vi "ExNframeBigBufNoDisplay.vi"() -> ()   [LabVIEW 2010]
uses:
  Open-Close Hardware/CamHandle.vi
panel:
  in  "Path":path=path "C:/Users/Public/Documents/SItoolkit/LabVIEW/Data Files/nframe.spe"
  in  "Number of Images":u32=1000 min=1 step=1
  out "ready to \nstart":bool
  in  "Start collection":bool
  in  "Exposure":dbl=1e-05 min=0.0 step=1e-06 format="%.7f"
  out "error out":errorcluster
  in  "error in (no error)":errorcluster
  # "ExCircNframeBigBufNoDisplay:\nThis example collects,  and saves in \na .spe file the number of images selected. This \nexample requires the camera have circular \nbuffers capability. \nFirst this example creates an array of image \nhandles. It then collects data into this array.\nFinally it displays and saves all the images."
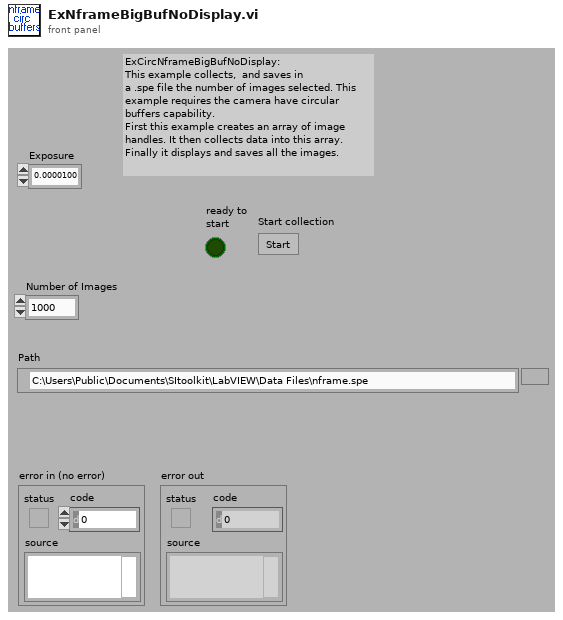
[diagram p1: front panel]
types:
  T1 = cluster{"acquire focus mode":u32, "Exposure":dbl, "Number of Images":u32, "Software accumulation":u32}
  T2 = cluster{"Camera Handle":u32, "Pulser Handle":u32, "File Handle":u32, "Display Handle":u32, "Image Handle":u32}
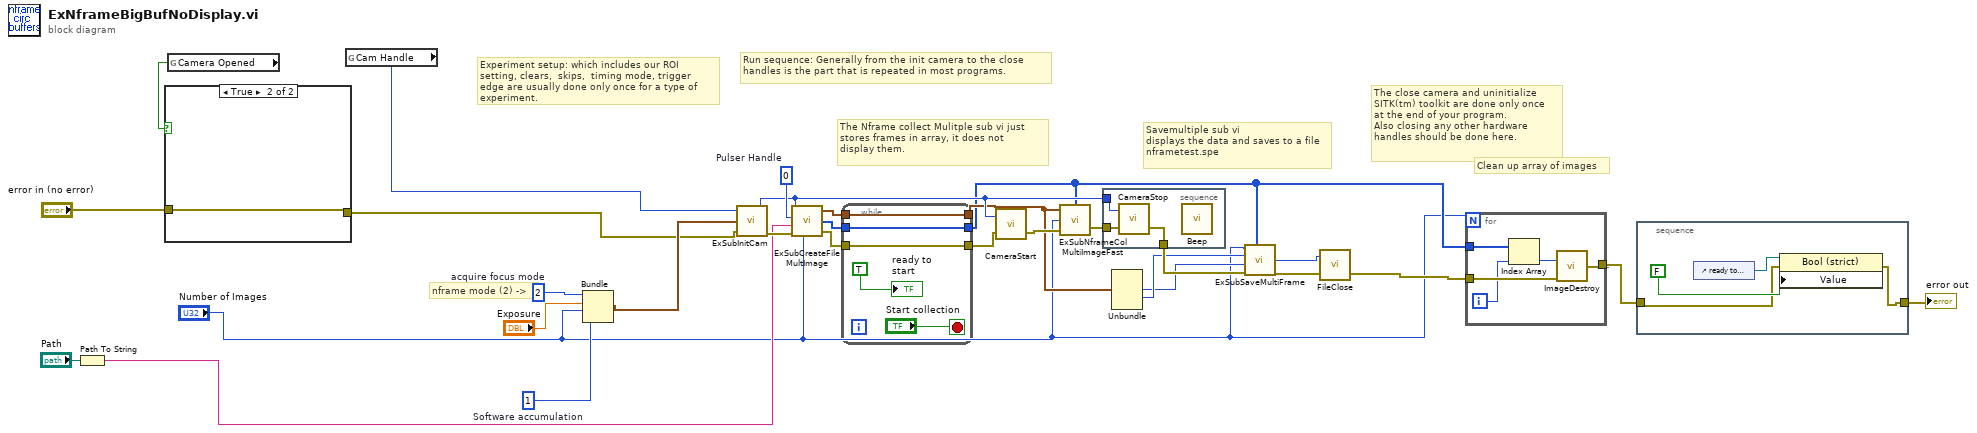
[diagram p0: block diagram]
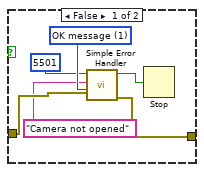
[diagram p2: hidden frame]
diagram:
  w26 = u32 0  # Pulser Handle
  w28 = u32 2  # acquire focus mode
  w27 = u32 1  # Software accumulation
  # "Clean up array of images"
  # "Savemultiple sub vi\ndisplays the data and saves to a file\nnframetest.spe"
  # "The Nframe collect Mulitple sub vi just \nstores frames in array, it does not \ndisplay them."
  # "The close camera and uninitialize\nSITK(tm) toolkit are done only once\nat the end of your program.\nAlso closing any other hardware \nhandles should be done here."
  # "Run sequence: Generally from the init camera to the close \nhandles is the part that is repeated in most programs."
  # "Experiment setup: which includes our ROI setting, clears,  skips,  timing mode, trigger edge are usually done only once for a type of experiment."
  # "nframe mode (2) ->"
  n1 = Path To String(path="Path") -> (string=w2:string)
  n2 = global read "CamHandle.vi" "Camera Opened"() -> (w9:bool)
  n3 = case shown="True" w9 {
    tunnel: "error in (no error)" -> [w35 w37]
    tunnel: [w34 w37] -> w5
    frame False {
      w36 = u16 1 items=["no dialog", "OK message", "continue or stop message"] ("type of dialog (OK msg:1)")
      n4 = call <vilib>:"Simple Error Handler.vi"("error code (no error:0)"=5501, "error source (\" \")"="Camera not opened", "type of dialog (OK msg:1)"=w36, "error in (no error)"=w35) -> ("error?"=w32:bool, "error out"=w34:errorcluster)  [unwired: 1 in, 3 out]
      n5 = Stop(stop? (T)=w32) -> ()
    }
    frame True {
    }
  }
  n6 = global read "CamHandle.vi" "Cam Handle"() -> (w4:u32)
  n7 = Bundle("acquire focus mode"=w28, "Exposure"="Exposure", "Number of Images"="Number of Images", "Software accumulation"=w27) -> (w6:T1)  [unwired: 1 in]
  n8 = call "ExSubInitCam.vi"("error in (no error)"=w5, "Camera Information"=w6, "Camera Handle"=w4) -> ("error out"=w29:errorcluster, "Camera Handle"=w23:u32)
  n9 = call "ExSubCreateFileMultImage.vi"("Camera Handle"=w23, "Pulser Handle"=w26, "File and Display Name"=w2, "error in (no error)"=w29, "Number of Images"="Number of Images") -> ("Handles Out"=w17:T2, "Array"=w13:u32[], "error out"=w15:errorcluster)
  n10 = while {
    tunnel: w17 -> [w42]
    tunnel: [w42] -> w16
    tunnel: w15 -> [w41]
    tunnel: [w41] -> w14
    tunnel: w13 -> [w40]
    tunnel: [w40] -> w12
    stop <- "Start collection" stop-if-true
    "ready to \nstart" <- TRUE
  }
  n11 = call <userlib>:"CameraStart.vi"("error in"=w14, "Camera Handle"=w23) -> ("error out"=w25:errorcluster)  [unwired: 1 out]
  n12 = call "ExSubNframeColMultiImageFast.vi"("image handles"=w12, "error in (no error)"=w25, "Number of Images"="Number of Images", "Handle Cluster"=w16) -> ("error out"=w24:errorcluster)  [unwired: 1 out]
  n13 = stacked-sequence {
    tunnel: w24 -> [w45]
    tunnel: w23 -> [w44]
    tunnel: [w43] -> w22
    frame #0 {
      n14 = call <userlib>:"CameraStop.vi"("error in"=w45, "Camera Handle"=w44) -> ("error out"=w43:errorcluster)  [unwired: 1 out]
      n15 = call <vilib>:"Beep.vi"() -> ()  [unwired: 12 in]
    }
  }
  n16 = Unbundle(w16) -> ("File Handle"=w20:u32, "Display Handle"=w21:u32)  [unwired: 3 out]
  n17 = call "ExSubSaveMultiFrame.vi"("Number of Images"="Number of Images", "Display Handle"=w21, "file handle"=w20, "error in (no error)"=w22, "Data handles"=w12) -> ("file Handle"=w18:u32, "error out"=w19:errorcluster)  [unwired: 1 out]
  n18 = call <userlib>:"FileClose.vi"("error in"=w19, "File Handle"=w18) -> ("error out"=w7:errorcluster)
  n19 = for {
    N: "Number of Images" -> [_]
    tunnel: w7 -> [w50]
    tunnel: [w49] -> w11
    tunnel: w12 -> [w47]
    i -> [w48]
    n20 = Index Array(array=w47, index=w48) -> (element=w46:u32)
    n21 = call <userlib>:"ImageDestroy.vi"("error in"=w50, "Data handle"=w46) -> ("error out"=w49:errorcluster)
  }
  n22 = stacked-sequence {
    tunnel: w11 -> [w52]
    tunnel: [w51] -> w8
    frame #0 {
      n23 = control-ref of="ready to \nstart"() -> (w54:refnum<vi>)
      n24 = property class="Bool (strict)"(reference=w54, error in=w52, "Value"=FALSE) -> (error out=w51:errorcluster)  [unwired: 1 out]
    }
  }
  "error out" <- w8
